vi "SetUSB5AoSampleRate.vi"(8 "错误输入（无错误）":errorcluster, 9 "SamplePeriod(ns)":u32=10000, 10 "Chan":u8, 11 "DevIndex":i32) -> (0 "错误输出":errorcluster, 3 "DevIndex Out":i32)   [LabVIEW 2020]
uses:
  lib/x64/USB5000.dll
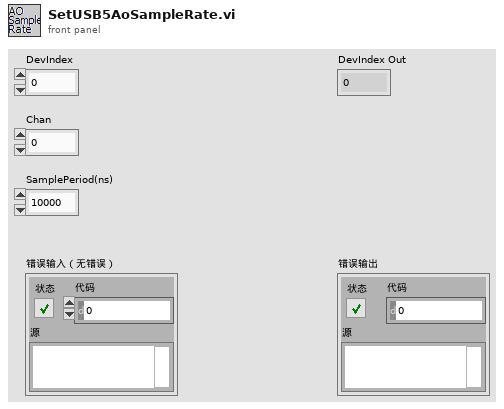
[diagram p1: front panel]
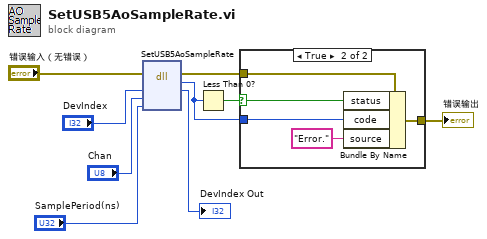
[diagram p0: block diagram]
diagram:
  n1 = dll-call lib="C:/Users/phosense/Downloads/USB-5000/USB-5000_LabVIEW/lib/x64/USB5000.dll" fn="SetUSB5AoSampleRate"(error in="错误输入（无错误）", "DevIndex"="DevIndex", "Chan"="Chan", "SamplePeriod"="SamplePeriod(ns)") -> (error out=w3:errorcluster, "返回类型"=w2:i32, "DevIndex"=→"DevIndex Out":i32)  [unwired: 4 in, 1 out]
  n2 = Less Than 0?(x=w2) -> (x < 0?=w4:bool)
  n3 = case shown="True" w4 {
    selector: w4 -> [_ w11]
    tunnel: [w10 w13] -> w1
    tunnel: w2 -> [_ w15]
    tunnel: w3 -> [w10 w12]
    frame False {
    }
    frame True {
      n4 = Bundle By Name(cluster=w12, "status"=w11, "code"=w15, "source"="Error." ("error message (\"\")")) -> (w13:errorcluster)
    }
  }
  "错误输出" <- w1
